vi "Write Lock-in.vi"(8 "error in (no error)":errorcluster, 10 "Lock-in":bool, 11 "Lock-in Command Msg in":refnum<class "Lock-in Command Msg.lvclass">) -> (0 "error out":errorcluster, 3 "Lock-in Command Msg out":refnum<class "Lock-in Command Msg.lvclass">)   [LabVIEW 2021, in "Lock-in Command Msg.lvclass"]
uses:
  Lock-in Command Msg.lvclass
  Lock-in Command Msg.lvclass/Lock-in Command Msg.ctl
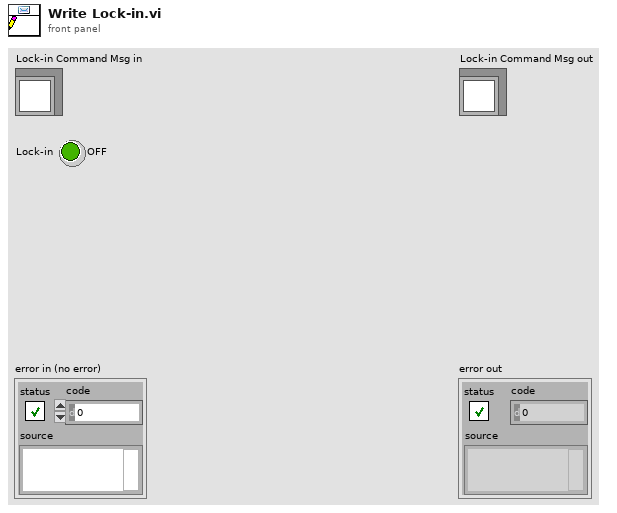
[diagram p1: front panel]
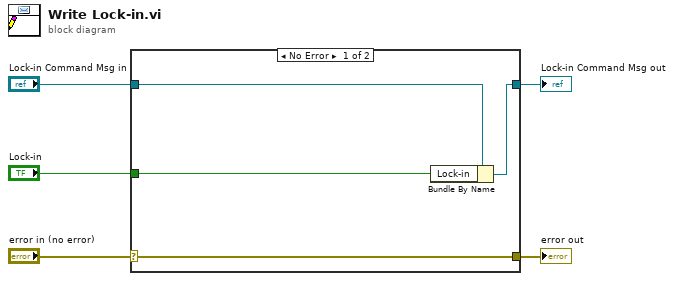
[diagram p0: block diagram]
diagram:
  n1 = case shown="No Error" "error in (no error)" {
    selector: "error in (no error)" -> [w9 w10]
    tunnel: [w9 w10] -> w4
    tunnel: [w7 w11] -> w2
    tunnel: "Lock-in Command Msg in" -> [w8 w11]
    tunnel: "Lock-in" -> [w6 _]
    frame No Error {
      n2 = Bundle By Name(cluster=w8, "Lock-in"=w6) -> (w7:refnum<class "Lock-in Command Msg.lvclass">)
    }
    frame Error {
    }
  }
  "error out" <- w4
  "Lock-in Command Msg out" <- w2
